vi "Initialise Gyroscope.vi"(8 "error in (no error)":errorcluster, 11 "LSM9DS1 IMU in":refnum<class "LSM9DS1 IMU.lvclass">) -> (0 "error out":errorcluster, 3 "LSM9DS1 IMU out":refnum<class "LSM9DS1 IMU.lvclass">)   [LabVIEW 2020, in "LSM9DS1 IMU.lvclass"]
uses:
  LSM9DS1 IMU.lvclass
  LSM9DS1 IMU.lvclass/LSM9DS1 IMU.ctl
  Read Accel & Gyro I2C.vi
  Write Accel & Gyro I2C.vi
  LINX I2C/LINX I2C.lvclass
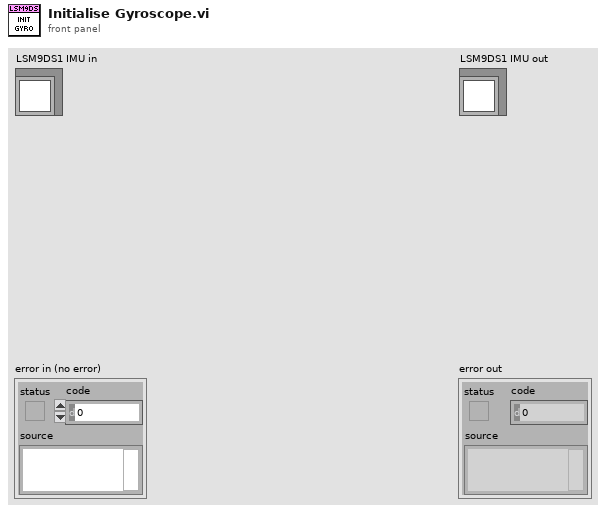
[diagram p1: front panel]
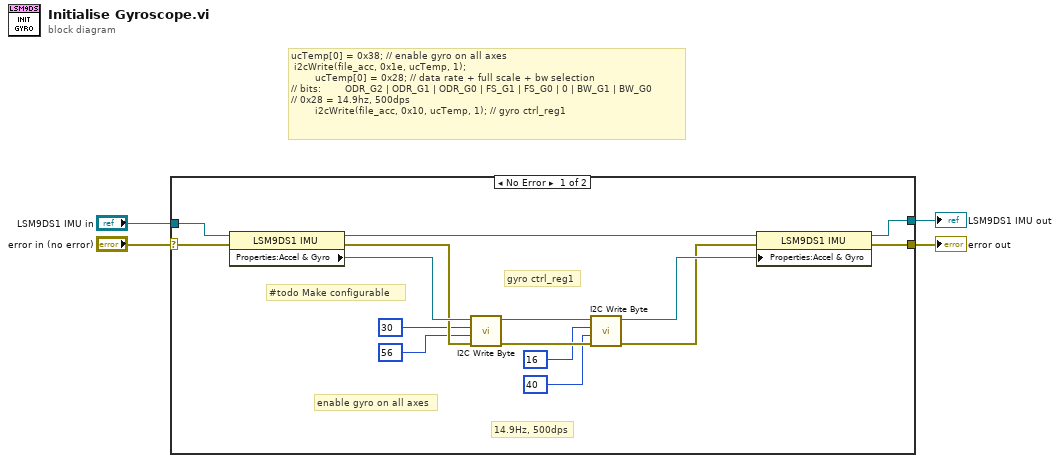
[diagram p0: block diagram]
diagram:
  # "ucTemp[0] = 0x38; // enable gyro on all axes\n\ti2cWrite(file_acc, 0x1e, ucTemp, 1);\n        ucTemp[0] = 0x28; // data rate + full scale + bw selection\n// bits:        ODR_G2 | ODR_G1 | ODR_G0 | FS_G1 | FS_G0 | 0 | BW_G1 | BW_G0\n// 0x28 = 14.9hz, 500dps\n        i2cWrite(file_acc, 0x10, ucTemp, 1); // gyro ctrl_reg1"
  n1 = case shown="No Error" "error in (no error)" {
    selector: "error in (no error)" -> [w14 w21]
    tunnel: [w13 w21] -> w3
    tunnel: [w16 w20] -> w1
    tunnel: "LSM9DS1 IMU in" -> [w19 w20]
    frame No Error {
      # "14.9Hz, 500dps"
      # "gyro ctrl_reg1"
      # "enable gyro on all axes"
      # "#todo Make configurable"
      n2 = property class="LSM9DS1 IMU"(reference=w19, error in=w14) -> (reference out=w17:refnum<class "LSM9DS1 IMU.lvclass">, error out=w15:errorcluster, "Properties:Accel & Gyro"=w18:refnum<class "LINX I2C.lvclass">)
      n3 = call "I2C Write Byte.vi"("error in (no error)"=w15, "Value"=u8 56 ("I2C Slave Address 2"), "Register Address"=u8 30 ("I2C Slave Address 2"), "LINX I2C in"=w18) -> ("error out"=w8:errorcluster, "LINX I2C out"=w12:refnum<class "LINX I2C.lvclass">)  [unwired: 6 in]
      n4 = call "I2C Write Byte.vi"("error in (no error)"=w8, "Value"=u8 40 ("I2C Slave Address 2"), "Register Address"=u8 16 ("I2C Slave Address 2"), "LINX I2C in"=w12) -> ("error out"=w7:errorcluster, "LINX I2C out"=w11:refnum<class "LINX I2C.lvclass">)  [unwired: 6 in]
      n5 = property class="LSM9DS1 IMU"(reference=w17, error in=w7, "Properties:Accel & Gyro"=w11) -> (reference out=w16:refnum<class "LSM9DS1 IMU.lvclass">, error out=w13:errorcluster)
    }
    frame Error {
    }
  }
  "error out" <- w3
  "LSM9DS1 IMU out" <- w1
